vi "Log External Data.vi"(11 "External Data TD":T1) -> ()   [LabVIEW 2016]
uses:
  External data TD.ctl
  <vilib>/Utility/file.llb/Write Delimited Spreadsheet (string).vi
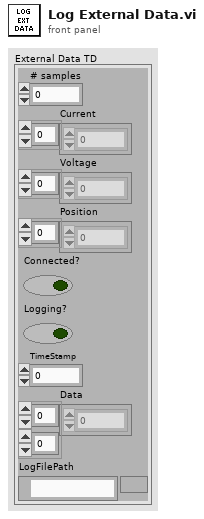
[diagram p1: front panel]
types:
  T1 = typedef "External data TD.ctl" = cluster{"# samples":i32, "Current":dbl[], "Voltage":dbl[], "Position":dbl[], "Connected?":bool, "Logging?":bool, "TimeStamp":dbl, "Data":dbl[][], "LogFilePath":path}
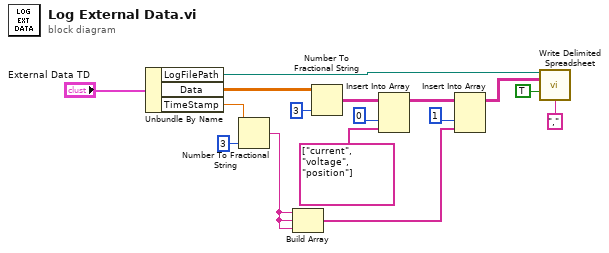
[diagram p0: block diagram]
diagram:
  n1 = Unbundle By Name("External Data TD") -> ("LogFilePath"=w16:path, "Data"=w12:dbl[][], "TimeStamp"=w6:dbl)
  n2 = Number To Fractional String(number=w6, precision (6)=i16 3) -> (F-format string=w5:string)  [unwired: 2 in]
  n3 = Build Array(w5, w5, w5) -> (w1:string[])
  n4 = Number To Fractional String(number=w12, precision (6)=i16 3) -> (F-format string=w11:string[][])  [unwired: 2 in]
  n5 = Insert Into Array(array=w11, index (col)=0 ("index (row)"), new element=string[] ["current", "voltage", "position"]) -> (w3:string[][])  [unwired: 1 in]
  n6 = Insert Into Array(array=w3, index (col)=1 ("index (row)"), new element=w1) -> (w4:string[][])  [unwired: 1 in]
  n7 = call-poly <vilib>:"Write Delimited Spreadsheet.vi"("file path (dialog if empty)"=w16, "2D data"=w4, "append to file? (new file:F)"=TRUE, "delimiter (\\t)"="," ("delimiter (\\t)")) -> ()  [unwired: 10 in, 2 out]
